vi "Create.vi"(8 "error in (no error)":errorcluster, 10 "VI:s to Measure":path[](array[path])) -> (0 "error out":errorcluster, 3 "Coverage Report":refnum<class "Coverage Report.lvclass">)   [LabVIEW 2020, in "Coverage Report.lvclass"]
uses:
  Coverage Report.lvclass
  Coverage Report.lvclass/Coverage Report.ctl
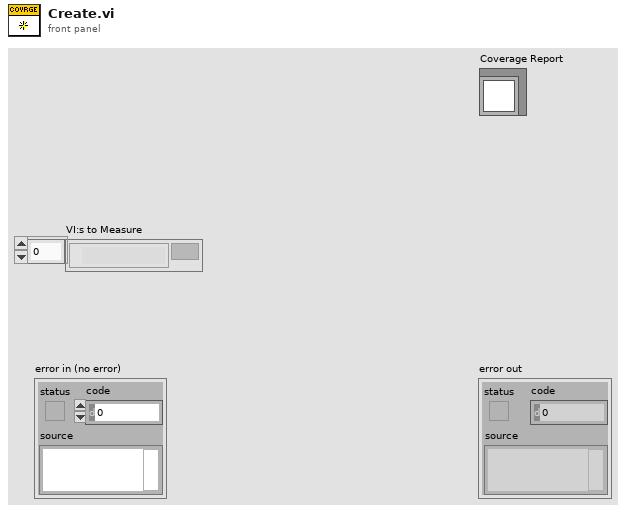
[diagram p1: front panel]
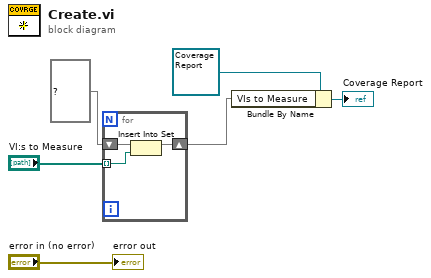
[diagram p0: block diagram]
diagram:
  n1 = for {
    tunnel: "VI:s to Measure" -> [w7] mode=indexing
    shift-right: [w8] -> w2
    shift-left: set{path} {} ("VIs to Measure") -> [w9]
    n2 = Insert Into Set(10:w7, 11:w9) -> (3:w8:set{path})  [unwired: 1 out]
  }
  n3 = Bundle By Name(cluster=refnum<class "Coverage Report.lvclass"> refnum ("Coverage Report"), "VIs to Measure"=w2) -> (→"Coverage Report":refnum<class "Coverage Report.lvclass">)
  "error out" <- "error in (no error)"
